vi "Error Handling.vi"(7 "error in (no error)":errorcluster, 11 "return type":i32) -> (8 "error out":errorcluster={"status"=FALSE, "code"=0, "source"="No Error"}, 15 "Error?":bool)   [LabVIEW 2014]
doc: "Converts the DLL Error Codes to LabVIEW Error Codes. \nYou can change the offset of the numeric codes here."
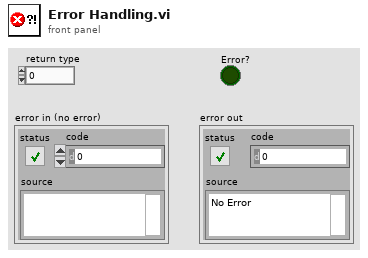
[diagram p1: front panel]
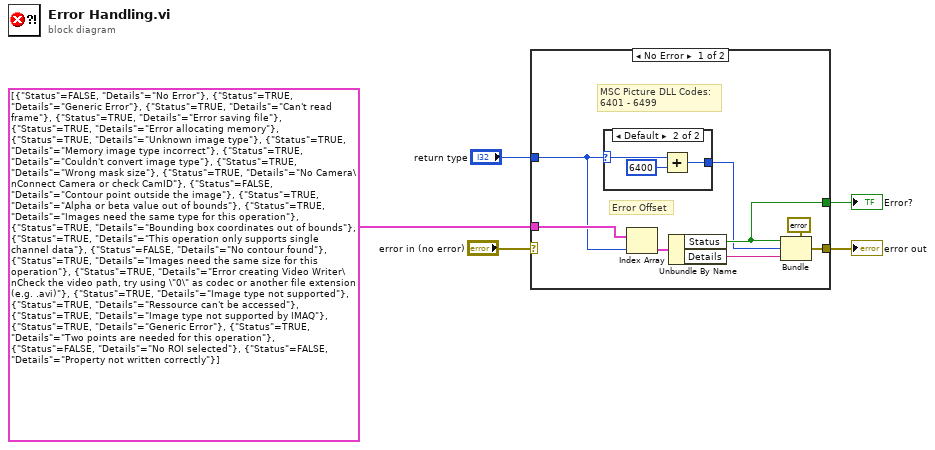
[diagram p0: block diagram]
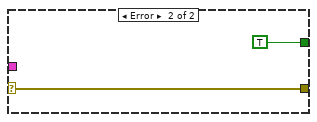
[diagram p3: hidden frame]
diagram:
  n1 = case shown="No Error" "error in (no error)" {
    selector: "error in (no error)" -> [_ w19]
    tunnel: "return type" -> [w10 _]
    tunnel: [w13 w19] -> w4
    tunnel: cluster{"Status":bool, "Details":string}[] [{"Status"=FALSE, "Details"="No Error"}, {"Status"=TRUE, "Details"="Generic Error"}, {"Status"=TRUE, "Details"="Can't read frame"}, {"Status"=TRUE, "Details"="Error saving file"}, {"Status"=TRUE, "Details"="Error allocating memory"}, {"Status"=TRUE, "Details"="Unknown image type"}, {"Status"=TRUE, "Details"="Memory image type incorrect"}, {"Status"=TRUE, "Details"="Couldn't convert image type"}, {"Status"=TRUE, "Details"="Wrong mask size"}, {"Status"=TRUE, "Details"="No Camera\nConnect Camera or check CamID"}, {"Status"=FALSE, "Details"="Contour point outside the image"}, {"Status"=TRUE, "Details"="Alpha or beta value out of bounds"}, {"Status"=TRUE, "Details"="Images need the same type for this operation"}, {"Status"=TRUE, "Details"="Bounding box coordinates out of bounds"}, {"Status"=TRUE, "Details"="This operation only supports single channel data"}, {"Status"=FALSE, "Details"="No contour found"}, {"Status"=TRUE, "Details"="Images need the same size for this operation"}, {"Status"=TRUE, "Details"="Error creating Video Writer\nCheck the video path, try using \"0\" as codec or another file extension (e.g. .avi)"}, {"Status"=TRUE, "Details"="Image type not supported"}, {"Status"=TRUE, "Details"="Ressource can't be accessed"}, {"Status"=TRUE, "Details"="Image type not supported by IMAQ"}, {"Status"=TRUE, "Details"="Generic Error"}, {"Status"=TRUE, "Details"="Two points are needed for this operation"}, {"Status"=FALSE, "Details"="No ROI selected"}, {"Status"=FALSE, "Details"="Property not written correctly"}] -> [w11 _]
    tunnel: [w12 TRUE ("Status")] -> w1
    frame No Error {
      # "Error Offset"
      # "MSC Picture DLL Codes:\n6401 - 6499"
      n2 = case shown="Default" w10 {
        selector: w10 -> [w14 w17]
        tunnel: [w14 w15] -> w7
        frame ..0 {
        }
        frame Default {
          n3 = Add(x=w17, y=u64 6400) -> (x+y=w15:u64)
        }
      }
      n4 = Index Array(array=w11, index=w10) -> (element=w9:cluster{"Status":bool, "Details":string})
      n5 = Unbundle By Name(w9) -> ("Status"=w12:bool, "Details"=w6:string)
      n6 = Bundle(cluster=errorcluster {"status"=FALSE, "code"=0, "source"=""} ("error in"), "status"=w12, "code"=w7, "source"=w6) -> (w13:errorcluster)
    }
    frame Error {
    }
  }
  "error out" <- w4
  "Error?" <- w1
